vi "Move to grid demo 2014 .vi"() -> ()   [LabVIEW 2014]
panel:
  out "Running":bool
  in  "Y angle":dbl(slide)=-0.19999999999999835 min=-30.0 max=30.0 step=0.1 scale=-30.0..30.0
  in  "X angle":dbl(slide)=-0.39999999999999836 min=-30.0 max=30.0 step=0.1 scale=-30.0..30.0
  out "error out":errorcluster
  in  "stop":bool
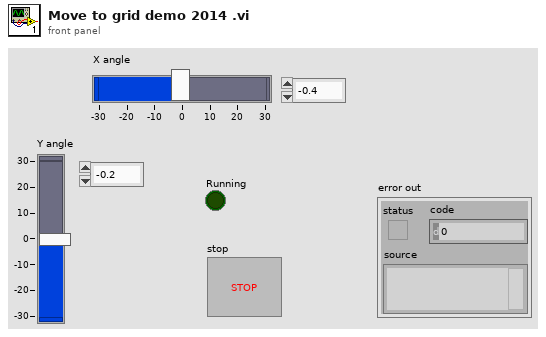
[diagram p1: front panel]
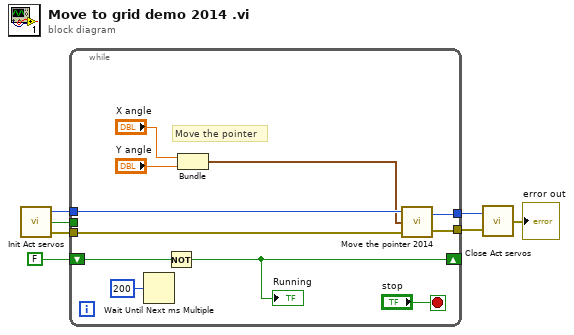
[diagram p0: block diagram]
diagram:
  n1 = call "Init Act servos.vi"() -> ("Device Out"=w2:i32, "Engaged?"=w4:bool, "error out"=w3:errorcluster)  [unwired: 1 in]
  n2 = while {
    tunnel: w2 -> [w14]
    tunnel: w3 -> [w13]
    tunnel: w4 -> [_]
    tunnel: [w18] -> w5
    tunnel: [w17] -> w6
    shift-right: [w9] -> _
    shift-left: FALSE -> [w10]
    stop <- "stop" stop-if-true
    # "Move the pointer"
    n3 = Wait Until Next ms Multiple(millisecond multiple=u32 200) -> ()  [unwired: 1 out]
    n4 = Not(x=w10) -> (.not. x?=w9:bool)
    "Running" <- w9
    n5 = Bundle("X angle"="X angle", "Y angle"="Y angle") -> (w8:cluster{"X angle":dbl, "Y angle":dbl})  [unwired: 1 in]
    n6 = call "Move the pointer 2014.vi"("error in (no error)"=w13, "Servo Angles"=w8, "Device In"=w14) -> ("error out"=w17:errorcluster, "Device Out"=w18:i32)
  }
  n7 = call "Close Act servos.vi"("error in"=w6, "Device In"=w5) -> ("error out"=→"error out":errorcluster)
